vi "Parse Sting.vi"(9 "Enum":T1, 10 "regular expression":string, 11 "String":string) -> (1 "Sinking":string[](array[string]), 2 "Sourcing":string[](array[string]), 3 "Parsed String":string)   [LabVIEW 2010]
uses:
  Typedef Command List.ctl
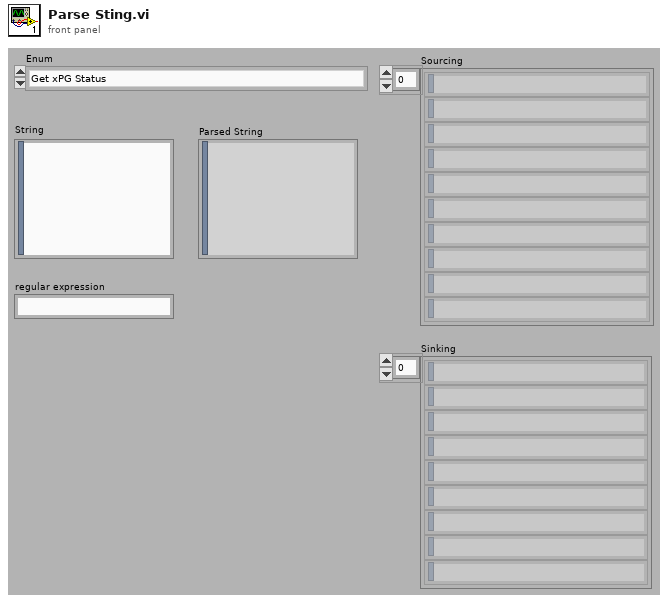
[diagram p1: front panel]
types:
  T1 = typedef "Typedef Command List.ctl" = enum16{"Get xPG Status", "xPG Stimulation", "Select Program", "Increment Program Amplitude", "Decrement Program Amplitude", "Get PoP Constants", "Get PPC Constants", "Get Program Names", "Set Pulse Amplitude", "Increment Pulse Amplitude", "Decrement Pulse Amplitude", "Get Pulse Widths", "Set Pulse Widths", "Increment Pulse Width", "Decrement Pulse Width", "Get Program Frequency", "Set Program Frequency", "Increment Program Frequency", "Decrement Program Frequency", "Inject Event", "Charging Control", "Get xPG Identity", "Set xPG Identity", "Restore Program Defaults", "Get Program Definition", "Set Program Definition", "Get Program Constants", "Set Program Constants", "Get Configurable Device Parameters", "Set Configurable Device Parameters", "Get Pulse Constants", "Set Pulse Constants", "Get Lead Limits", "Set Lead Limits", "Get Channel Calibrations", "Set Channel Calibrations", "<reserved 2>", "<reserved 3>", "<reserved 4>", "<reserved 5>", "<reserved 6>", "<reserved 7>", "Get Stim Asic HV Calibrations", "Set Stim Asic HV Calibrations", "<reserved 8>", "<reserved 9>", "Get CP Data", "Set CP Data", "Clear Log", "Read Log", "Append Log", "Get Patient Program Runtime", "Set Patient Program Runtime", "Impedance Measurement", "Enter Storage Mode", "Echo Short", "Echo Long", "Get General Calibration", "Set General Calibration", "Get Trim List", "Set Trim List", "Get Counter", "Set Counter", "Get Test Stimulation", "Set Test Stimulation", "Get Titration Stimulation", "Set Titration Stimulation", "Get Ramp Time", "Set Ramp Time", "Get VBAT", "Set Software Description Block", "Get Software Description Block", "Write Memory", "Read Memory", "Reset xPG", "Erase Flash Block", "Write Vectors", "Read Vectors", "Diagnostic Data", "Set Background Impedance", "Get Background Impedence ", "Set Test Waveform", "Calibrate Channel", "Get Log Range", "Reserved 0x55", "Reserved 0x56", "MICS Options", "Pair PPC", "Pair POP", "Stop Bootloader", "Tune MICS", "MICS Diagnostics", "Undefined"}
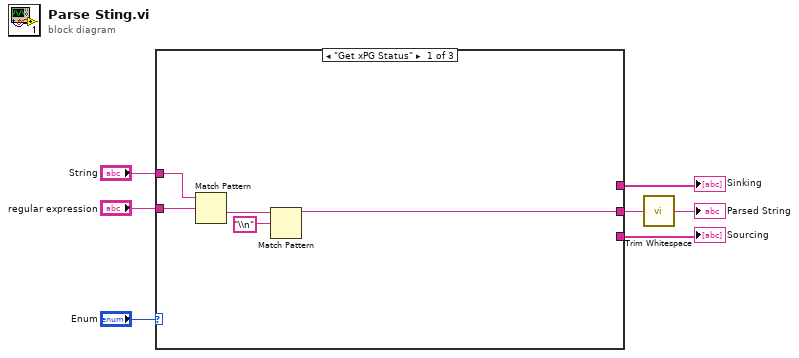
[diagram p0: block diagram]
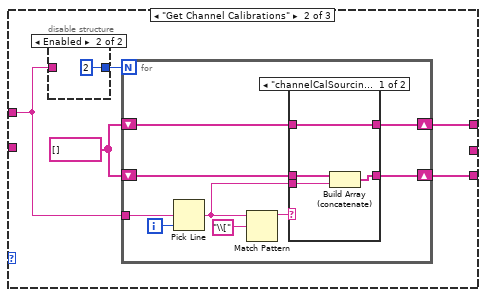
[diagram p2: hidden frame]
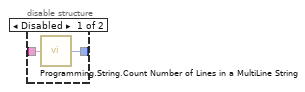
[diagram p3: hidden frame]
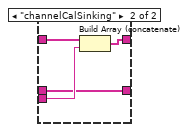
[diagram p4: hidden frame]
diagram:
  n1 = case shown="\"Get xPG Status\"" "Enum" {
    tunnel: "String" -> [w10 w15 _]
    tunnel: "regular expression" -> [w9 _ _]
    tunnel: [_ w14 _] -> w4
    tunnel: [_ w13 _] -> w3
    tunnel: [w8 _ _] -> w2
    frame "Get xPG Status" {
      n2 = Match Pattern(string=w10, regular expression=w9) -> (after substring=w12:string)  [unwired: 1 in, 3 out]
      n3 = Match Pattern(string=w12, regular expression="\\n") -> (before substring=w8:string)  [unwired: 1 in, 3 out]
    }
    frame "Get Channel Calibrations" {
      w17 = string[] []
      n4 = disable-structure shown="Enabled" {
        disable-tunnel: [w19 2 ("Number of Lines")] -> w16
        disable-tunnel: w15 -> [w18 _]
        frame Disabled {
          n5 = call "Programming.String.Count Number of Lines in a MultiLine String.vi"("MultiLine String Input"=w18) -> ("Number of Lines"=w19:i32)  [unwired: 4 in]
        }
        frame Enabled {
        }
      }
      n6 = for {
        N: w16 -> [_]
        tunnel: w15 -> [w28]
        shift-right: [w22] -> w13
        shift-left: w17 -> [w25]
        shift-right: [w24] -> w14
        shift-left: w17 -> [w23]
        i -> [w27]
        n7 = Pick Line(multi-line string=w28, line index=w27) -> (output string=w26:string)  [unwired: 1 in]
        n8 = Match Pattern(string=w26, regular expression="\\[" ("format string")) -> (before substring=w21:string)  [unwired: 1 in, 3 out]
        n9 = case shown="\"channelCalSourcing\", Default" w21 {
          tunnel: w26 -> [w33 w37]
          tunnel: [w30 w36] -> w24
          tunnel: w25 -> [w32 w34]
          tunnel: w23 -> [w30 w35]
          tunnel: [w31 w34] -> w22
          frame "channelCalSourcing", Default {
            n10 = Build Array (concatenate)(w32, w33) -> (w31:string[])
          }
          frame "channelCalSinking" {
            n11 = Build Array (concatenate)(w35, w37) -> (w36:string[])
          }
        }
      }
    }
    frame Default {
    }
  }
  "Sourcing" <- w3
  "Sinking" <- w4
  n12 = call <vilib>:"Trim Whitespace.vi"("string"=w2) -> ("trimmed string"=→"Parsed String":string)  [unwired: 1 in]
